vi "Init.vi"(7 "I2C #":T2=-1, 8 "error in (no error)":errorcluster, 10 "Session In":refnum<class "Session.lvclass">, 11 "Address":T1=54 format="%02x") -> (0 "error out":errorcluster, 3 "AdaFruit-Seesaw out":refnum<class "AdaFruit-Seesaw.lvclass">)   [LabVIEW 2020, in "CTI-Peripheral.lvlib" / "AdaFruit-Seesaw.lvclass"]
uses:
  AdaFruit-Seesaw.lvclass
  CTI/Session/Session.lvclass
  CTI/I2C Number.ctl
  CTI/I2C Address.ctl
  CTI/I2C Connection/I2C Connection.lvclass/I2C Connection.ctl
  AdaFruit-Seesaw.lvclass/AdaFruit-Seesaw.ctl
  CTI/I2C Connection/I2C Connection.lvclass
  CTI/CTI.lvlib
panel:
  out "Date":u16
  out "Version":u16
  out "HW_ID":string
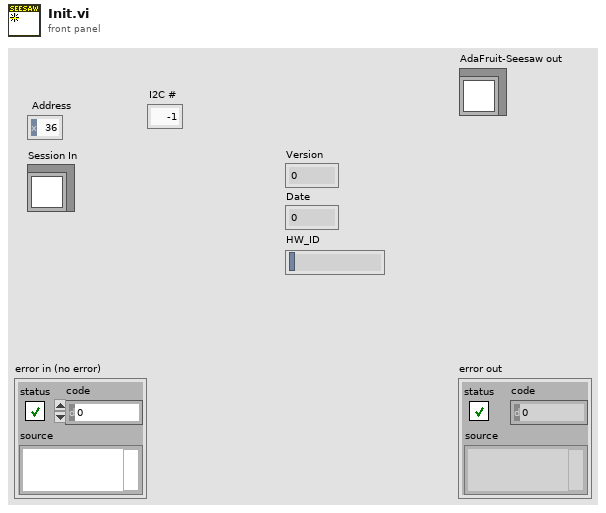
[diagram p1: front panel]
types:
  T1 = typedef "CTI.lvlib/I2C Address.ctl" = u8
  T2 = typedef "CTI.lvlib/I2C Number.ctl" = i8
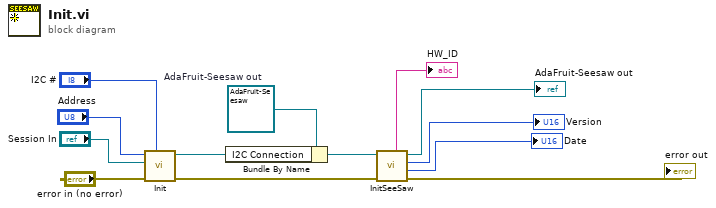
[diagram p0: block diagram]
diagram:
  w11 = refnum<class "AdaFruit-Seesaw.lvclass"> refnum  # AdaFruit-Seesaw out
  n1 = call "Init.vi"("I2C #"="I2C #", "error in (no error)"="error in (no error)", "Session"="Session In", "Address"="Address") -> ("error out"=w6:errorcluster, "I2C Connection"=w13:refnum<class "I2C Connection.lvclass">)  [unwired: 6 in]
  n2 = Bundle By Name(cluster=w11, "I2C Connection"=w13) -> (w7:refnum<class "AdaFruit-Seesaw.lvclass">)
  n3 = call "InitSeeSaw.vi"("error in (no error)"=w6, "AdaFruit-Seesaw in"=w7) -> ("error out"=→"error out":errorcluster, "Date"=→"Date":u16, "Version"=→"Version":u16, "AdaFruit-Seesaw out"=→"AdaFruit-Seesaw out":refnum<class "AdaFruit-Seesaw.lvclass">, "HW_ID"=→"HW_ID":string)  [unwired: 5 in]
